vi "FPGA_Lock-In_PID.vi"() -> ()   [LabVIEW 2012]
panel:
  out "Reference Output":dbl
  out "P+I Error":dbl
  in  "Integral Gain":dbl
  in  "Proportional Gain":ext
  out "PID Input Error":dbl
  in  "PID Stop":bool
  out "Phase (Rad) Shift Difference":dbl
  in  "Phase Control":dbl
  out "Partial Phase":dbl
  out "Phase (Degree) Shift Difference":dbl
  out "P1":dbl
  out "P2":dbl
  out "Signal Output":dbl
  out "Filtered Signal":dynamicdata(graph)
  out "Multiplication of Signals":dynamicdata(graph)
  in  "Lock-In Stop":bool
  out "Freq":dbl
  out "Amp_Signal":dbl
  out "Freq":dbl
  out "Amp_Ref":dbl
  # "Reference Signal"
  # "Input Signal"
  # "PID Microcontroller"
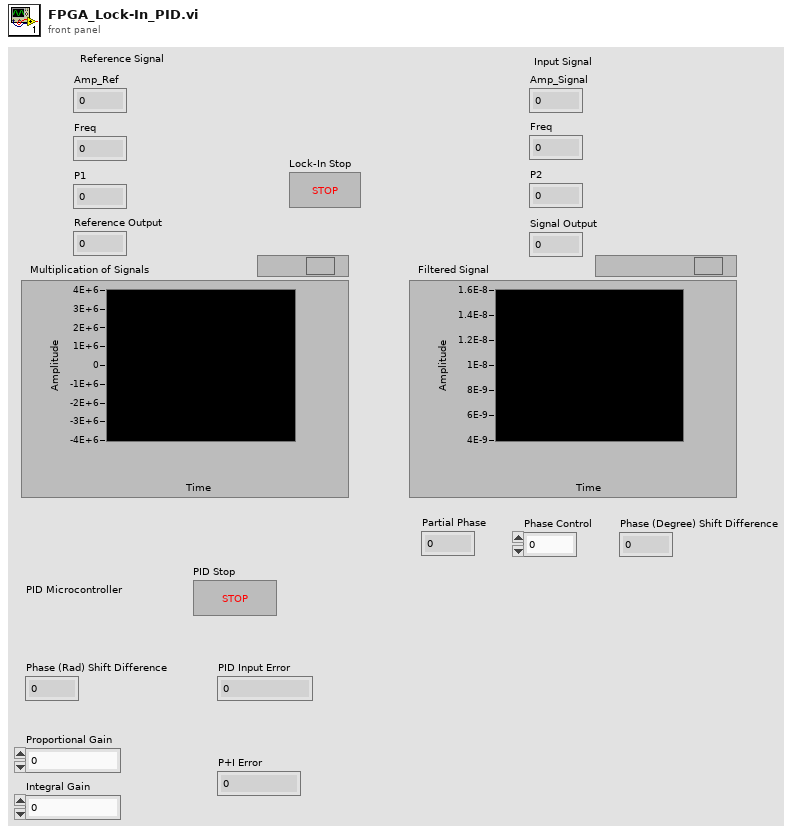
[diagram p1: front panel]
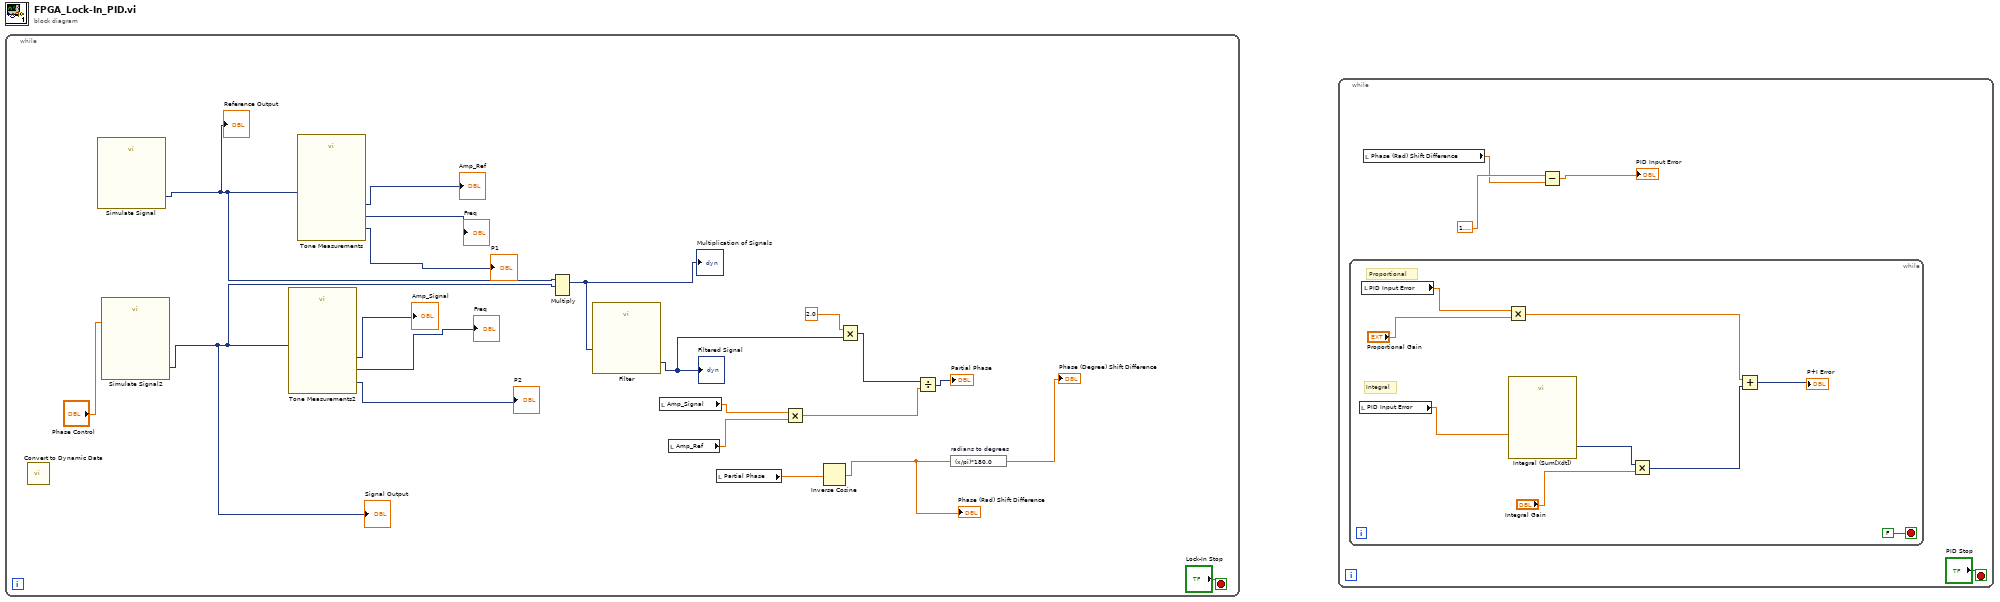
[diagram p0: block diagram]
diagram:
  n1 = while {
    stop <- "Lock-In Stop" stop-if-true
    n2 = call "Convert to Dynamic Data"() -> ()  [unwired: 4 in, 1 out]
    n3 = call "Simulate Signal"() -> ("Sine"=w1:dynamicdata)  [unwired: 14 in, 1 out]
    "Reference Output" <- w1
    n4 = call "Simulate Signal2"("Phase"="Phase Control") -> ("Sine"=w15:dynamicdata)  [unwired: 13 in, 1 out]
    "Signal Output" <- w15
    n5 = call "Tone Measurements2"("Signals"=w15) -> ("Phase"=→"P2":dynamicdata, "Frequency"=→"Freq":dynamicdata, "Amplitude"=→"Amp_Signal":dynamicdata)  [unwired: 7 in, 1 out]
    n6 = call "Tone Measurements"("Signals"=w1) -> ("Phase"=→"P1":dynamicdata, "Frequency"=→"Freq":dynamicdata, "Amplitude"=→"Amp_Ref":dynamicdata)  [unwired: 7 in, 1 out]
    n7 = Multiply(1:w15, 2:w1) -> (0:w16:dynamicdata)  [unwired: 1 in, 1 out]
    "Multiplication of Signals" <- w16
    n8 = call "Filter"("Signal"=w16) -> ("Filtered Signal"=w11:dynamicdata)  [unwired: 9 in, 1 out]
    "Filtered Signal" <- w11
    n9 = local read "Amp_Signal"() -> (w10:dbl)
    n10 = local read "Amp_Ref"() -> (w9:dbl)
    n11 = local read "Partial Phase"() -> (w5:dbl)
    n12 = Multiply(x=w10, y=w9) -> (x*y=w7:dbl)
    n13 = Inverse Cosine(1:w5) -> (0:w2:dbl)
    "Phase (Rad) Shift Difference" <- w2
    n14 = Multiply(x=2.0, y=w11) -> (x*y=w8:dynamicdata)
    n15 = Divide(x=w8, y=w7) -> (x/y=→"Partial Phase":dynamicdata)
    n16 = expression code="(x/pi)*180.0" "radians to degrees"(w2) -> (→"Phase (Degree) Shift Difference":dbl)
  }
  n17 = while {
    stop <- "PID Stop" stop-if-true
    n18 = while {
      stop <- FALSE stop-if-true
      # "Integral"
      # "Proportional"
      n19 = local read "PID Input Error"() -> (w31:dbl)
      n20 = local read "PID Input Error"() -> (w33:dbl)
      n21 = Multiply(x=w33, y="Proportional Gain") -> (x*y=w28:ext)
      n22 = call "Integral (Sum[Xdt])"("Signals"=w31) -> ("Result"=w30:dynamicdata)  [unwired: 5 in, 1 out]
      n23 = Multiply(x=w30, y="Integral Gain") -> (x*y=w27:dynamicdata)
      n24 = Add(x=w28, y=w27) -> (x+y=→"P+I Error":dynamicdata)
    }
    n25 = local read "Phase (Rad) Shift Difference"() -> (w22:dbl)
    n26 = Subtract(x=1.5707963267948966, y=w22) -> (x-y=→"PID Input Error":dbl)
  }
